vi "labview_client.vi"() -> ()   [LabVIEW 2019]
panel:
  out "error out":errorcluster
  out "data out":string
  in  "stop":bool
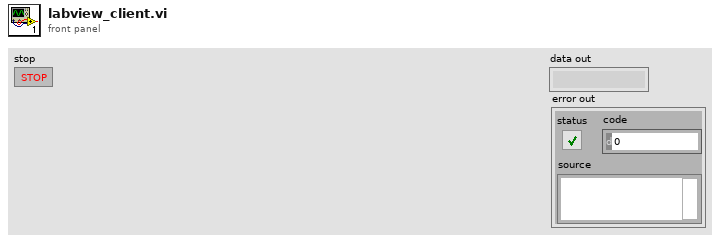
[diagram p1: front panel]
types:
  T1 = enum16{"Standard", "Buffered", "CRLF", "Immediate"}
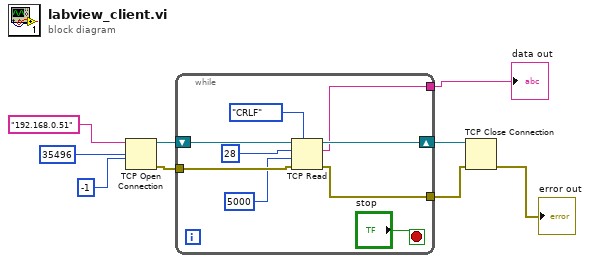
[diagram p0: block diagram]
diagram:
  n1 = TCP Open Connection(address="192.168.0.51", remote port or service name=u16 35496, timeout ms (60000)=-1) -> (connection ID=w9:refnum<k5>, error out=w4:errorcluster)  [unwired: 2 in]
  n2 = while {
    shift-right: [w17] -> w8
    shift-left: w9 -> [w18]
    tunnel: w4 -> [w13]
    tunnel: [w12] -> w3
    tunnel: [w11] -> w1
    stop <- "stop" stop-if-true
    n3 = TCP Read(connection ID=w18, bytes to read=28, error in (no error)=w13, 7:T1."CRLF" ("mode (standard)"), 9:5000 ("timeout ms (25000)")) -> (connection ID out=w17:refnum<k5>, data out=w11:string, error out=w12:errorcluster)
  }
  "data out" <- w1
  n4 = TCP Close Connection(connection ID=w8, error in (no error)=w3) -> (error out=→"error out":errorcluster)  [unwired: 1 in, 1 out]
